vi "CS_Start.vi"() -> ()   [LabVIEW 2014]
doc: "\"Main\" of a CS system on the local machine. Mailny the SuperProc should be started from here. Other objects are created by the SuperProc itself. A list of names of all the objects to be created by the user is part of the data base (SuperProc->Special0-SpecialN).\n\nLicense Agreement for this software:\n\nCopyright (C) 2013 Holger Brand, Dennis Neidherr\nGSI Helmholtzzentrum für Schwerionenforschung GmbH\nPlanckstraße 1\nD-64291 Darmstadt\nGermany\n\nContact: d.neidherr@gsi.de \n\nThis program is free software: you can redistribute it and/or modify it under the terms\nof the GNU General Public License as published by the Free Software Foundation, either\nversion 3 of the License, or (at your option) any later version.\n\nThis program is distributed in the hope that it will be useful, but WITHOUT ANY WARRANTY;\nwithout even the implied warranty of MERCHANTABILITY or FITNESS FOR A PARTICULAR PURPOSE.\nSee the GNU General Public License for more details.\n\nYou should have received a copy of the GNU General Public License along with this program.\nIf not, see <http://www.gnu.org/licenses/>.\n\nFor all questions and ideas contact: d.neidherr@gsi.de or h.brand@gsi.de\nLast update: 20-Mar-2013\n\nmenuHelpStart\nFile\n==\n- \"Shutdown\" gently exits the CS system by removing all objects\n- \"Exit\" unfriendly exits the CS system by exiting the application without removing of objects. \n\nTools\n===\n- \"UserGOG\" displays a generic object GUI (GOG) for on-line testing purposes by the user sitting in front of the computer. If you would like to routinely open a GOG when a CS system starts, please configure a dedicated GOG via the database and configure the SuperProc to create that GOG upon starting up the system.\n\n- \"Inspector\" shows information on the objects of THIS and other CS systems.\n\n- \"DIM Table\" provides a simple possibility for viewing DIM services.\n\n- \"DIM Trend\" can be used for trending of DIM services\n\n- \"DIM Histogram\" can be used for histogramming of multiple DIM services\n\n- \"Access Viewer\" can be used to view the hierarchy of reserved objects. Moreover, it allows for locking the access to certain objects and sub-systems.\n\n- \"DSC Alarm Viewer\" is the alarm viewer of the SCADA backend based on the LabVIEW DSC module. When using the alarm viewer, you will be asked for the name of the DSC interface. The alarm viewer requires a binary compiled with the CSDSC_SCADA package.\nmenuHelpStop\n\ndescriptionHelpStart\n\"Main\" of a CS instance. CS is a framework that can be used by many experiments. CS is a multi-threaded, event driven, object oriented and distributed framework with SCADA functionality. An experiment control system can be developed by combining the CS framework with experiment specific add-ons.\n\nMore information available at http://wiki.gsi.de/cgi-bin/view/CSframework\n\ndescriptionHelpStop"
uses:
  CSClass/CSCore/GUIs/GOGFrontPanel/GOGFrontPanel.i attribute.ctl
  CSClass/CSCore/BaseProcess/BaseProcess.descriptor string definition.ctl
  CSClass/CSCore/CSSystem/CSSystemLib/CSSystemLib.instances options.ctl
  CSlibraries-extern/DimLVEvent/LVDimInterface/LVDimInterface.dim service type.ctl
  CSlibraries/UtilityLib/UtilityLib.helpType.ctl
  CSClass/CSCore/CSSystem/CoreDefs/CoreDefs.error_severity.ctl
  CSClass/CSCore/CSSystem/CoreDefs/CoreDefs.error_type.ctl
  CSlibraries/UtilityLib/UtilityLib.valueStatus.ctl
  CSlibraries-extern/DimLVEvent/LVDimInterface/LVDimInterface.dic_info_service_notifier.vi
  CSClass/CSCore/CSSystem/CoreLib/CoreLib.lvlib
  CSlibraries-extern/DimLVEvent/LVDimInterface/LVDimInterface.lvlib
  CSClass/CSCore/CSSystem/CSSystemLib/CSSystemLib.lvlib
  CSClass/CSCore/BaseProcess/BaseProcess.lvlib
  CSlibraries/UtilityLib/UtilityLib.lvlib
  CSClass/CSCore/CSObj/CSObj.lvlib
  CSClass/CSCore/CAEObj/CAEObj.lvlib
  CSClass/CSCore/BaseSM/BaseSM.lvlib
  CSClass/CSCore/BaseGUI/BaseGUI.lvlib
  CSClass/CSCore/GUIs/GOGFrontPanel/GOGFrontPanel.lvlib
panel:
  in  "False":bool
  out "database":string="Process@"
  out "domainInfo":string="hello world :-)"
  in  "GOGFrontPanel.i attribute":T1
  out "system running":bool=TRUE
  out "status":string="shutting down..."
  out "systemID":string="TestSystem@KSTest@lxgs11.gsi.de"
  out "error out":errorcluster
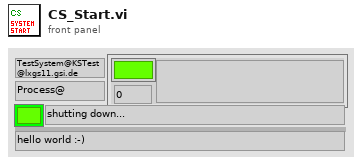
[diagram p1: front panel]
types:
  T1 = typedef "GOGFrontPanel.lvlib/GOGFrontPanel.i attribute.ctl" = cluster{"GOGObject":string, "Object":string, "Method":string, "Descriptor":T2, "Input Descriptor":string, "Output Descriptor":string, "inputNames":string[], "outputNames":string[], "Values":cluster{"descriptor":string, "value":string}[]}
  T2 = typedef "BaseProcess.lvlib/BaseProcess.descriptor string definition.ctl" = string
  T3 = enum32{"Invalid", "Standard", "Closed", "Hidden", "Minimized", "Maximized"}
  T4 = enum32{"invalid app kind", "Development System", "Run Time System", "Student Edition", "Embedded LabVIEW", "Evaluation", "Custom"}
  T5 = typedef "CSSystemLib.lvlib/CSSystemLib.instances options.ctl" = enum16{"add", "delete", "name2ref", "ref2name ", "ref2class", "obj exists?", "cleanup", "get I list", "get I list all", "ref2myclasses", "setClassNames"}
  T6 = enum16{"acquire queue", "release queue", "destroy queue", "get command ID", "destroy all queues"}
  T7 = typedef "UtilityLib.lvlib/UtilityLib.helpType.ctl" = enum16{"unknown", "menu", "description", "about", "special0", "special1", "special2"}
  T8 = typedef "CoreDefs.error_type.ctl" = enum16{"no error", "can't load process", "can't unload process", "process does not exist", "can't install process", "can't remove process", "unknown function", "time out", "can't execute function", "duplicate queue name", "super not found", "caller queue invalid", "can't ping process", "unknown error", "VISA Error", "VISA timeout", "GPIB timeout", "GPIB error", "communication error", "data type mismatch", "can't read data from OPC server", "can't write data to OPC server", "OET error", "function not implemented", "process already exists", "invalid Shared Variable name", "error writing Shared Variable", "error reading Shared Variable", "invalid client name", "corrupt database", "unknown class", "call not authorized", "parameter out of range", "OET timeout: can't get data to modify", "invalid queue name", "requested operation incompatible with current state", "event undefined", "event disabled", "state undefined", "caller is not a friend", "EventBuilder: bad eventID", "EventBuilder: no DAQ devices", "a thread must not stop itself", "UNUSED ELEMENT4", "DiscArchiver: eventData incomplete", "DiscArchiver: eventData does not belong to run", "DiscArchiver: can't open file", "DiscArchiver: can't write to file", "DiscArchiver: available disc space low", "can't acquire semaphore", "error reading data from database", "notifier object is not existing", "can't register process", "can't unregister process", "illegal event type", "object disabled", "object already exists", "can't change state", "Instrument not found", "no connection to remote node", "invalid reference", "N/A", "UNUSED ELEMENT 1", "element not found", "illegal TCP/IP connection detected", "object does not exist", "invalid access ID", "unknown CS system", "invalid privilige", "unsupported data type", "unsupported server type", "IO server already exists", "Shared Variable already exists"}
  T9 = typedef "CoreDefs.error_severity.ctl" = enum16{"undefined", "information", "warning", "error", "fatal"}
  T10 = typedef "UtilityLib.lvlib/UtilityLib.valueStatus.ctl" = enum16{"no info available", "stand by/off", "on", "warning", "alarm/malfunction", "not implemented", "user action required", "important information", "system default", "control default", "indicator default", "button default"}
  T11 = enum32{"Bad", "Idle", "Run top level", "Running"}
  T12 = typedef "LVDimInterface.lvlib/LVDimInterface.dim service type.ctl" = u16
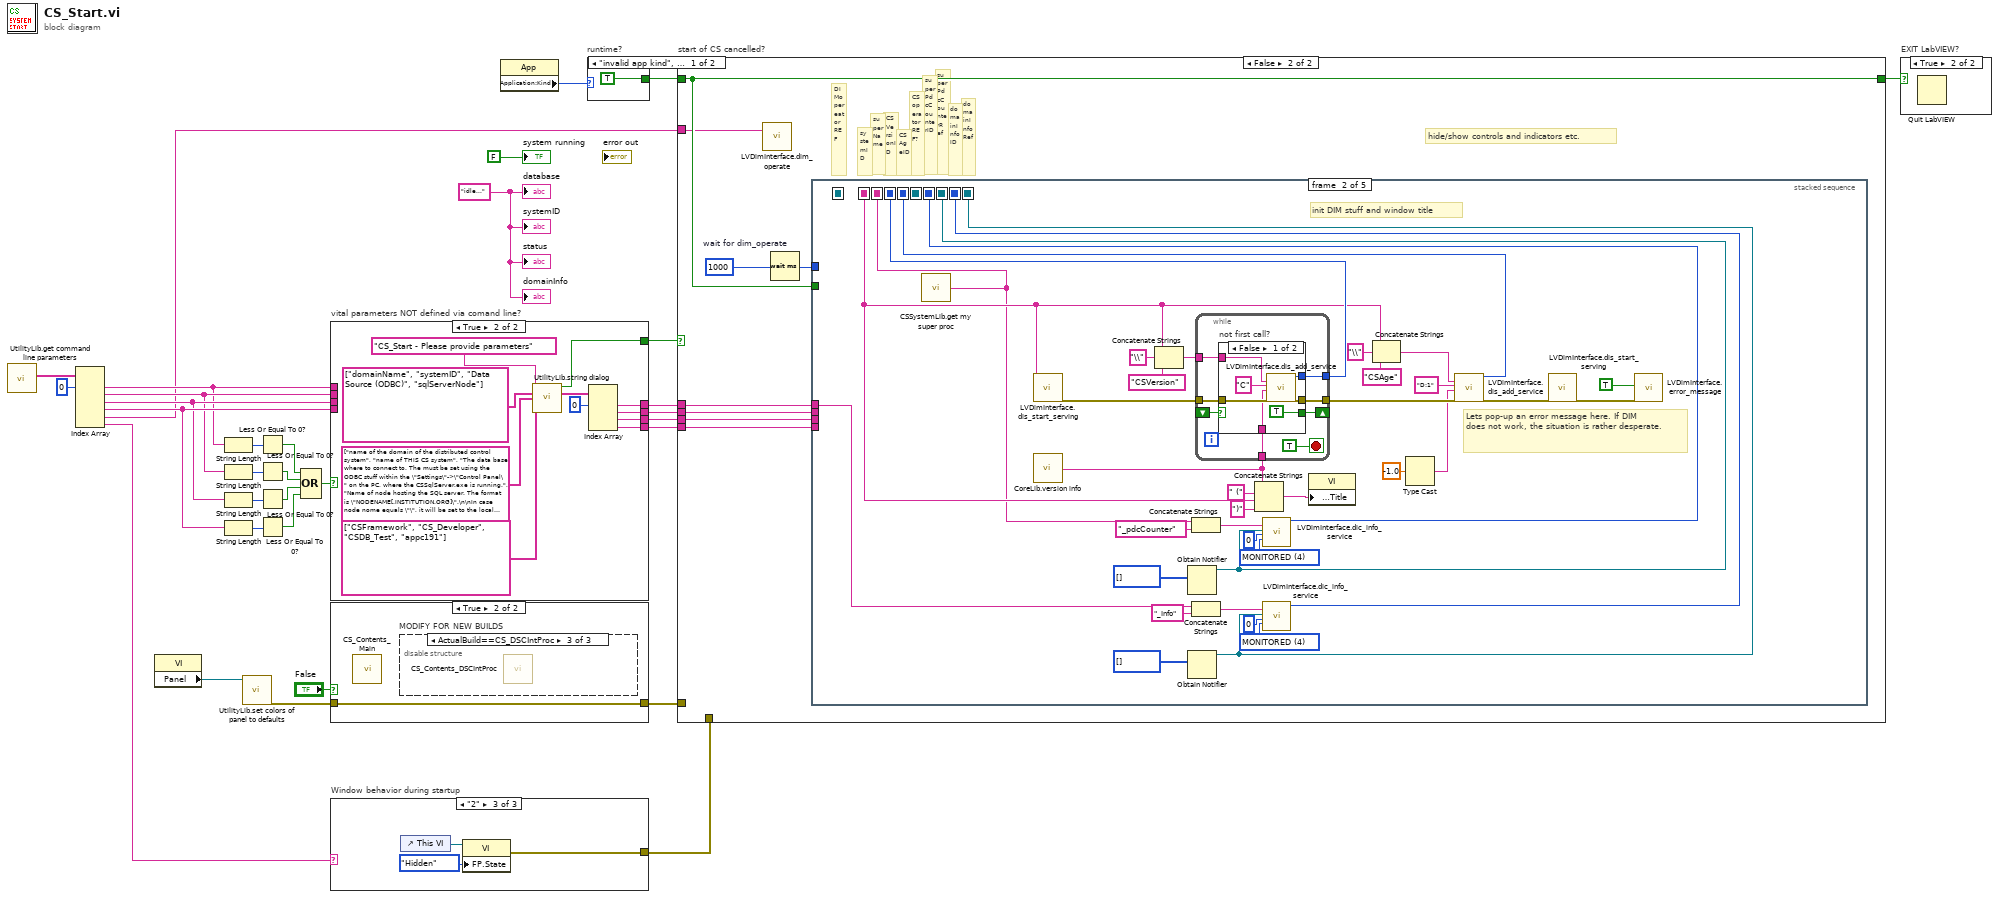
[diagram p0: block diagram]
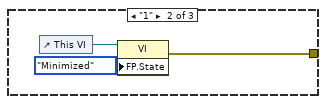
[diagram p3: hidden frame]
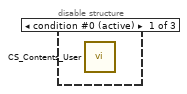
[diagram p5: hidden frame]
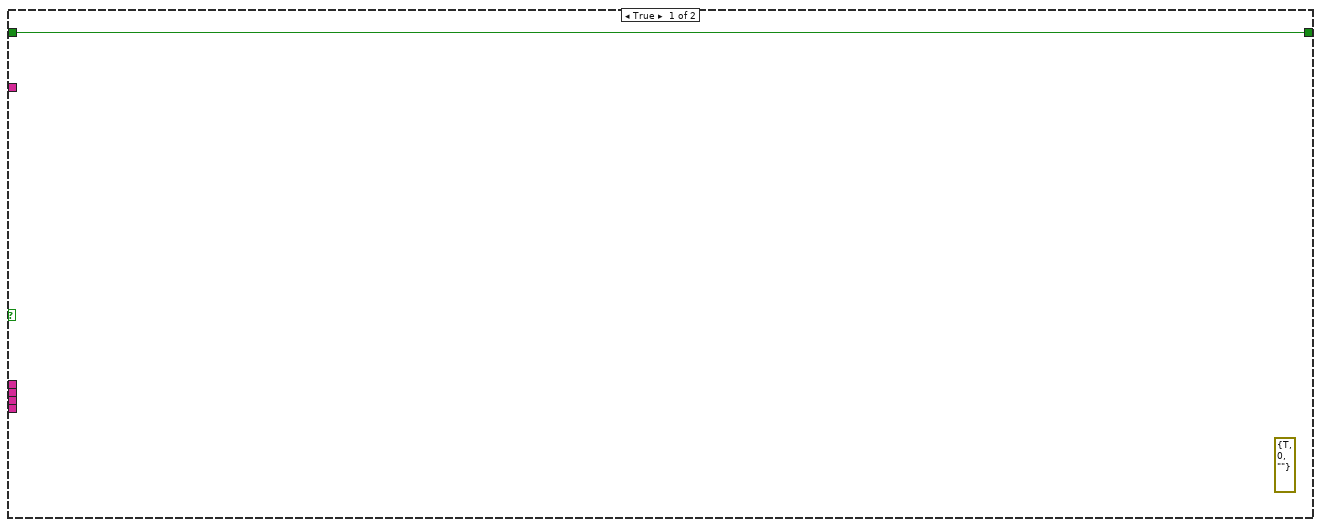
[diagram p8: hidden frame]
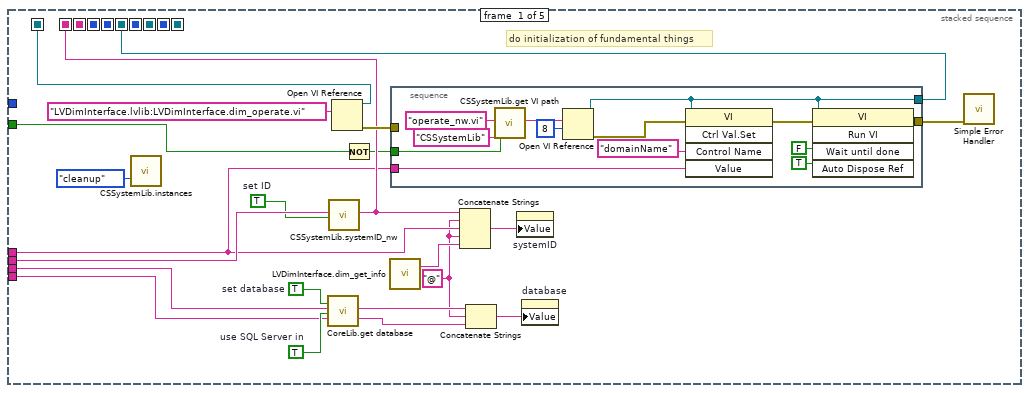
[diagram p9: hidden frame]
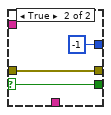
[diagram p10: hidden frame]
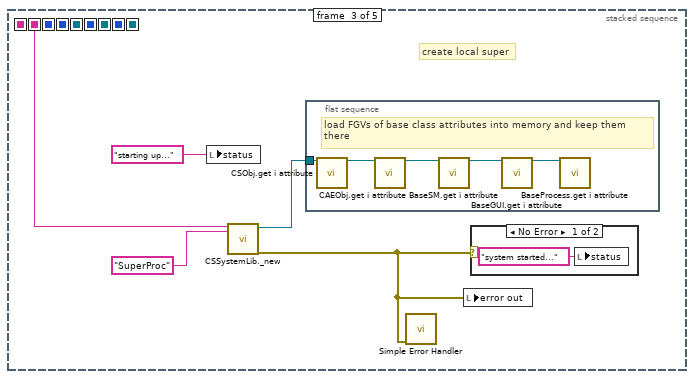
[diagram p11: hidden frame]
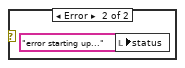
[diagram p12: hidden frame]
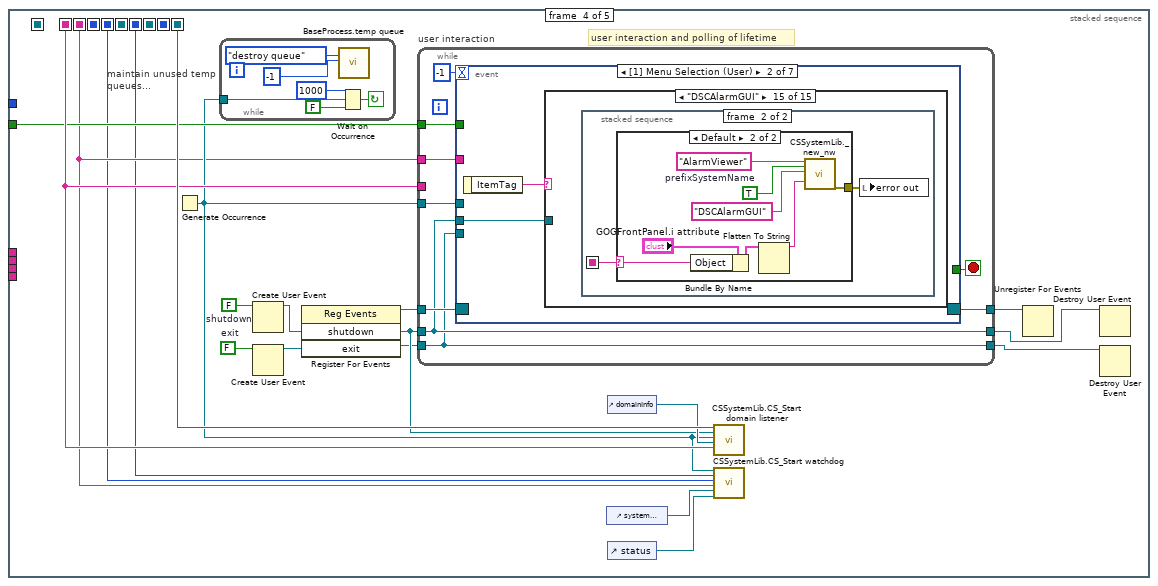
[diagram p13: hidden frame]
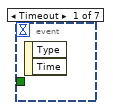
[diagram p14: hidden frame]
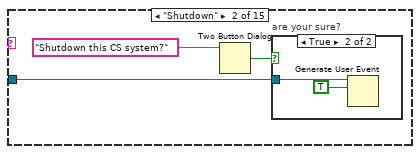
[diagram p16: hidden frame]
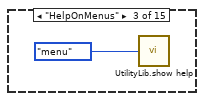
[diagram p18: hidden frame]
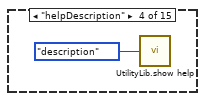
[diagram p19: hidden frame]
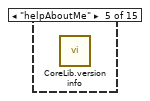
[diagram p20: hidden frame]
diagram:
  w10 = "idle..." ("status")
  n1 = call "UtilityLib.get command line parameters.vi"() -> ("parametersCleaned"=w30:string[])  [unwired: 9 in, 2 out]
  n2 = Index Array(array=w30, index #1=0 ("index")) -> (element #1=w18:string, element #2=w20:string, element #3=w22:string, element #4=w29:string, element #5=w5:string, element #6=w2:string)  [unwired: 5 in]
  n3 = property class="VI"() -> ("Panel"=w6:refnum<vi>)  [unwired: 2 in, 2 out]
  n4 = String Length(string=w18) -> (length=w17:i32)
  n5 = String Length(string=w20) -> (length=w19:i32)
  n6 = String Length(string=w22) -> (length=w21:i32)
  n7 = String Length(string=w29) -> (length=w27:i32)
  n8 = call "UtilityLib.set colors of panel to defaults.vi"("Front Panel"=w6) -> ("error out"=w9:errorcluster)  [unwired: 18 in]
  n9 = Less Or Equal To 0?(x=w17) -> (x <= 0?=w23:bool)
  n10 = Less Or Equal To 0?(x=w19) -> (x <= 0?=w24:bool)
  n11 = Less Or Equal To 0?(x=w21) -> (x <= 0?=w25:bool)
  n12 = Less Or Equal To 0?(x=w27) -> (x <= 0?=w28:bool)
  n13 = Compound Arithmetic op=OR(w23, w24, w25, w28) -> (w26:bool)
  n14 = case "vital parameters NOT defined via comand line?" shown="True" w26 {
    tunnel: [w36 w42] -> w14
    tunnel: w18 -> [w36 _]
    tunnel: [w35 w40] -> w1
    tunnel: w20 -> [w35 _]
    tunnel: w22 -> [w34 _]
    tunnel: [w34 w41] -> w13
    tunnel: w29 -> [w33 _]
    tunnel: [w33 w38] -> w12
    tunnel: [_ w39] -> w3
    frame False {
    }
    frame True {
      n15 = call "UtilityLib.string dialog.vi"("title"="CS_Start - Please provide parameters", "captions"=string[] ["domainName", "systemID", "Data Source (ODBC)", "sqlServerNode"], "helpText"=string[] ["name of the domain of the distributed control system", "name of THIS CS system", "The data base where to connect to. The must be set using the ODBC stuff within the \"Settings\"->\"Control Panel\" on the PC, where the CSSqlServer.exe is running.", "Name of node hosting the SQL server. The format is \"NODENAME[.INSTITUTION.ORG]\".\n\nIn case node nome equals \"\", it will be set to the local host."], "initialValue"=string[] ["CSFramework", "CS_Developer", "CSDB_Test", "appc191"]) -> ("cancelled"=w39:bool, "strings"=w44:string[])  [unwired: 8 in, 2 out]
      n16 = Index Array(array=w44, index #1=0 ("index")) -> (element #1=w42:string, element #2=w40:string, element #3=w41:string, element #4=w38:string)  [unwired: 3 in]
    }
  }
  n17 = case shown="True" "False" {
    tunnel: w9 -> [w48 w49]
    tunnel: [w48 w49] -> w8
    frame False {
    }
    frame True {
      n18 = call "CS_Contents_Main.vi"() -> ()  [unwired: 1 in]
      n19 = disable-structure "MODIFY FOR NEW BUILDS" shown="ActualBuild==CS_DSCIntProc" {
        frame condition #0 (active) {
          n20 = call "CS_Contents_User.vi"() -> ()  [unwired: 1 in]
        }
        frame condition #1 {
        }
        frame condition #2 {
          n21 = call "CS_Contents_DSCIntProc.vi"() -> ()  [unwired: 1 in]
        }
      }
    }
  }
  n22 = case "Window behavior during startup" shown="\"2\"" w2 {
    tunnel: [_ w52 w53] -> w4
    frame Default {
    }
    frame "1" {
      n23 = control-ref of="This VI"() -> (w50:refnum<vi>)
      n24 = property class="VI"(reference=w50, "FP.State"=T3."Minimized" ("Front Panel Window:State")) -> (error out=w52:errorcluster)  [unwired: 1 in, 1 out]
    }
    frame "2" {
      n25 = control-ref of="This VI"() -> (w55:refnum<vi>)
      n26 = property class="VI"(reference=w55, "FP.State"=T3."Hidden" ("Front Panel Window:State")) -> (error out=w53:errorcluster)  [unwired: 1 in, 1 out]
    }
  }
  n27 = property class="App"() -> ("Application:Kind"=w32:T4)  [unwired: 2 in, 2 out]
  n28 = case "runtime?" shown="\"invalid app kind\", Default" w32 {
    tunnel: [TRUE _] -> w16
    frame "invalid app kind", Default {
    }
    frame "Development System" {
    }
  }
  n29 = case "start of CS cancelled?" shown="False" w3 {
    tunnel: w16 -> [w57 w65]
    tunnel: [w57 w65] -> w15
    tunnel: w5 -> [_ w64]
    tunnel: w14 -> [_ w63]
    tunnel: w1 -> [_ w62]
    tunnel: w13 -> [_ w61]
    tunnel: w12 -> [_ w60]
    tunnel: w8 -> [_ _]
    tunnel: w4 -> [_ _]
    frame True {
      (unwired) errorcluster {"status"=TRUE, "code"=0, "source"=""} ("error out")
    }
    frame False {
      # "hide/show controls and indicators etc."
      # "domainInfoRef"
      # "domainInfoID"
      # "superPdcCounterRef"
      # "superPdcCounterID"
      # "CSoperator REF?"
      # "CSAgeID"
      # "CSVersionID"
      # "superName"
      # "systemID"
      # "DIMopereator REF"
      n30 = call "LVDimInterface.dim_operate.vi"("DNSNode"=w64) -> ()  [unwired: 19 in]
      n31 = Wait (ms) "wait for dim_operate"(milliseconds to wait=u32 1000) -> (millisecond timer value=w58:u32)
      n32 = stacked-sequence {
        seq-local: [w78 _ _ _ _] -> [_ w117 _ w184 _]
        seq-local: [w85 _ _ _ _] -> [_ _ _ _ w299]
        seq-local: [_ w109 _ _ _] -> [_ _ w158 w177 _]
        seq-local: [_ w126 _ _ _] -> [_ _ _ _ w295]
        seq-local: [_ w125 _ _ _] -> [_ _ _ w173 w294]
        seq-local: [w86 _ _ _ _] -> [_ _ _ _ w298]
        seq-local: [_ w113 _ _ _] -> [_ _ _ w174 w292]
        seq-local: [_ w112 _ _ _] -> [_ _ _ _ w290]
        seq-local: [_ w103 _ _ _] -> [_ _ _ _ w284]
        seq-local: [_ w102 _ _ _] -> [_ _ _ w185 w283]
        tunnel: w65 -> [w67 _ _ w180 w282]
        tunnel: w63 -> [w76 w101 _ _ _]
        tunnel: w62 -> [w77 _ _ _ _]
        tunnel: w61 -> [w81 _ _ _ _]
        tunnel: w60 -> [w80 _ _ _ _]
        tunnel: w58 -> [_ _ _ _ _]
        frame #0 {
          w74 = "@" ("string")
          w84 = TRUE  # use SQL Server in
          w87 = TRUE  # set database
          w66 = TRUE  # set ID
          # "do initialization of fundamental things"
          n33 = call "CSSystemLib.instances.vi"("Action"=CSSystemLib.instances_options."cleanup") -> ()  [unwired: 12 in, 7 out]
          n34 = call "CoreLib.get database.vi"("set database"=w87, "database in"=w81, "use SQL Server in"=w84, "SQL Server node in"=w80) -> ("database"=w75:string, "SQL Server node"=w73:string)  [unwired: 12 in, 2 out]
          n35 = call "CSSystemLib.systemID_nw.vi"("systemID"=w77, "Force set ID"=w66) -> ("systemID out"=w78:string)  [unwired: 16 in, 1 out]
          n36 = Open VI Reference(vi path="LVDimInterface.lvlib:LVDimInterface.dim_operate.vi") -> (vi reference=w85:refnum<vi>, error out=w82:errorcluster)  [unwired: 5 in]
          n37 = Not(x=w67) -> (.not. x?=w68:bool)
          n38 = call "LVDimInterface.dim_get_info.vi"() -> ("dimDnsNode"=w79:string)  [unwired: 13 in, 6 out]
          n39 = stacked-sequence {
            tunnel: w76 -> [w92]
            tunnel: [w96] -> w86
            tunnel: [w95] -> w69
            tunnel: w82 -> [_]
            tunnel: w68 -> [w89]
            frame #0 {
              n40 = call "CSSystemLib.get VI path.vi"("method"="operate_nw.vi" ("Method"), "class"="CSSystemLib" ("Class"), "reReead"=w89) -> ("VI path"=w91:string)  [unwired: 14 in, 2 out]
              n41 = Open VI Reference(vi path=w91, options=8) -> (vi reference=w96:refnum<vi>, error out=w99:errorcluster)  [unwired: 4 in]
              n42 = invoke class="VI" method="Ctrl Val.Set"(reference=w96, error in=w99, "Control Name"="domainName", "Value"=w92) -> (error out=w98:errorcluster)  [unwired: 1 in, 4 out]
              n43 = invoke class="VI" method="Run VI"(reference=w96, error in=w98, "Wait until done"=FALSE, "Auto Dispose Ref"=TRUE ("Auto Dispose Reference")) -> (error out=w95:errorcluster)  [unwired: 1 in, 4 out]
            }
          }
          n44 = Concatenate Strings(w78, w74, w76, w74, w79) -> (w72:string)
          n45 = Concatenate Strings(w75, w74, w73) -> (w71:string)
          n46 = property on="systemID" class="Str"("Value"=w72) -> ()  [unwired: 2 in, 2 out]
          n47 = property on="database" class="Str"("Value"=w71) -> ()  [unwired: 2 in, 2 out]
          n48 = call <vilib>:"Simple Error Handler.vi"("error in (no error)"=w69) -> ()  [unwired: 4 in, 5 out]
        }
        frame #1 {
          w108 = T12 4 items=["ONCE_ONLY"=1, "TIMED"=2, "MONITORED"=4] ("serviceType")
          w110 = T12 4 items=["ONCE_ONLY"=1, "TIMED"=2, "MONITORED"=4] ("serviceType")
          # "Lets pop-up an error message here. If DIM\ndoes not work, the situation is rather desperate."
          # "init DIM stuff and window title"
          n49 = call "CSSystemLib.get my super proc.vi"() -> ("name"=w109:string)  [unwired: 1 in]
          n50 = call "LVDimInterface.dis_start_serving.vi"("serverName"=w117) -> ("error out"=w134:errorcluster)  [unwired: 17 in, 1 out]
          n51 = call "CoreLib.version info.vi"() -> ("CS Version"=w121:string)  [unwired: 4 in, 1 out]
          n52 = Concatenate Strings(w117, "\\" ("string"), "CSVersion" ("string")) -> (w137:string)
          n53 = Obtain Notifier(notification data type=i8[] []) -> (notifier out=w112:refnum<notifier>)  [unwired: 3 in, 2 out]
          n54 = Obtain Notifier(notification data type=i8[] []) -> (notifier out=w102:refnum<notifier>)  [unwired: 3 in, 2 out]
          n55 = Concatenate Strings(w109, "_pdcCounter" ("string")) -> (w115:string)
          n56 = Concatenate Strings(w101, "_Info" ("string")) -> (w105:string)
          n57 = while {
            tunnel: w137 -> [w145]
            tunnel: w134 -> [w144]
            tunnel: [w143] -> w130
            tunnel: [w142] -> w126
            tunnel: w121 -> [w141]
            shift-right: [w139] -> _
            shift-left: _ -> [w138]
            stop <- TRUE stop-if-true
            n58 = case "not first call?" shown="False" w138 {
              selector: w138 -> [_ w153]
              tunnel: w145 -> [w152 _]
              tunnel: w144 -> [w150 w155]
              tunnel: [w149 w155] -> w143
              tunnel: [w148 -1 ("my_serviceID")] -> w142
              tunnel: w141 -> [w147 _]
              tunnel: [TRUE w153] -> w139
              frame False {
                n59 = call "LVDimInterface.dis_add_service.vi"("serviceName"=w152, "typeDescriptor"="C", "data"=w147, "error in (no error)"=w150) -> ("my_serviceID"=w148:i32, "error out"=w149:errorcluster)  [unwired: 14 in]
              }
              frame True {
              }
            }
          }
          n60 = Concatenate Strings(w121, " (" ("string"), w117, ")" ("string")) -> (w124:string)
          n61 = call-poly "LVDimInterface.dic_info_service.vi"("serviceName"=w115, "notifierRef"=w112, "timeout [s]"=0, "serviceType"=w110) -> ("callBackID"=w113:i32)  [unwired: 14 in, 1 out]
          n62 = call-poly "LVDimInterface.dic_info_service.vi"("serviceName"=w105, "notifierRef"=w102, "timeout [s]"=0, "serviceType"=w108) -> ("callBackID"=w103:i32)  [unwired: 14 in, 1 out]
          n63 = property class="VI"("Front Panel Window:Title"=w124) -> ()  [unwired: 2 in, 2 out]
          n64 = Concatenate Strings(w117, "\\" ("string"), "CSAge" ("string")) -> (w133:string)
          n65 = Type Cast(x=-1.0) -> (*(type *) &x=w128:string)  [unwired: 1 in]
          n66 = call "LVDimInterface.dis_add_service.vi"("serviceName"=w133, "typeDescriptor"="D:1", "data"=w128, "error in (no error)"=w130) -> ("my_serviceID"=w125:i32, "error out"=w119:errorcluster)  [unwired: 14 in]
          n67 = call "LVDimInterface.dis_start_serving.vi"("error in (no error)"=w119) -> ("error out"=w118:errorcluster)  [unwired: 17 in, 1 out]
          n68 = call "LVDimInterface.error_message.vi"("add message to source"=TRUE, "error in (no error)"=w118) -> ()  [unwired: 14 in, 4 out]
        }
        frame #2 {
          # "create local super"
          n69 = local write "status"("starting up..." ("status")) -> ()
          n70 = call "CSSystemLib._new.vi"("object name"=w158, "class name"="SuperProc") -> ("i ref out"=w157:refnum<vi>, "error out"=w156:errorcluster)  [unwired: 14 in, 2 out]
          n71 = flat-sequence {
            tunnel: w157 -> [w165]
            frame #0 {
              # "load FGVs of base class attributes into memory and keep them\nthere"
              n72 = call "CSObj.get i attribute.vi"("i ref in"=w165) -> ("i ref out"=w164:refnum<vi>)  [unwired: 16 in, 2 out]
              n73 = call "CAEObj.get i attribute.vi"("i ref in"=w164) -> ("i ref out"=w163:refnum<vi>)  [unwired: 16 in, 2 out]
              n74 = call "BaseSM.get i attribute.vi"("i ref in"=w163) -> ("i ref out"=w162:refnum<vi>)  [unwired: 16 in, 2 out]
              n75 = call "BaseGUI.get i attribute.vi"("i ref in"=w162) -> ("i ref out"=w161:refnum<vi>)  [unwired: 16 in, 2 out]
              n76 = call "BaseProcess.get i attribute.vi"("i ref in"=w161) -> ()  [unwired: 16 in, 3 out]
            }
          }
          n77 = call <vilib>:"Simple Error Handler.vi"("error in (no error)"=w156) -> ()  [unwired: 4 in, 5 out]
          n78 = local write "error out"(w156) -> ()
          n79 = case shown="No Error" w156 {
            frame No Error {
              n80 = local write "status"("system started..." ("status")) -> ()
            }
            frame Error {
              n81 = local write "status"("error starting up..." ("status")) -> ()
            }
          }
        }
        frame #3 {
          w171 = FALSE  # exit
          w172 = FALSE  # shutdown
          # "user interaction and polling of lifetime"
          n82 = Generate Occurrence() -> (w178:refnum<k4>)
          n83 = while "maintain unused temp queues..." {
            tunnel: w178 -> [w189]
            stop <- w190 continue-if-true
            n84 = Wait on Occurrence(1:FALSE ("ignore previous (T)"), 2:w189, 3:1000 ("ms timeout (-1)")) -> (0:w190:bool)
            n85 = call "BaseProcess.temp queue.vi"("Action"=T6."destroy queue", "ID in"=-1) -> ()  [unwired: 14 in, 4 out]
          }
          n86 = Create User Event(user event datatype=w172) -> (user event=w170:refnum<user-event>)  [unwired: 1 in, 1 out]
          n87 = Create User Event(user event datatype=w171) -> (user event=w169:refnum<user-event>)  [unwired: 1 in, 1 out]
          n88 = register-events(w170, w169) -> (reference out=w183:refnum<event-registration>)  [unwired: 2 in, 1 out]
          n89 = while "user interaction" {
            tunnel: w178 -> [w200]
            tunnel: w177 -> [w198]
            tunnel: w184 -> [_]
            tunnel: w180 -> [w196]
            tunnel: w183 -> [w195]
            tunnel: w170 -> [w194]
            tunnel: [w193] -> w182
            tunnel: [w194] -> w168
            tunnel: w169 -> [w192]
            tunnel: [w192] -> w181
            stop <- w199 stop-if-true
            n90 = event shown="[1] Menu Selection (User)" {
              selector: w195 -> [_ _ _ _ _ _ _]
              dyn-events: [_ _ _ _ _ _ _] -> w193
              timeout: -1 -> [_ _ _ _ _ _ _]
              tunnel: w200 -> [_ _ _ w265 _ _ _]
              tunnel: w198 -> [_ _ _ w264 _ _ _]
              tunnel: [_ _ _ w263 _ _ _] -> w199
              tunnel: w196 -> [_ _ _ _ _ _ w277]
              tunnel: w194 -> [_ w201 _ _ _ _ _]
              tunnel: w192 -> [_ _ _ _ w272 w276 _]
              event Timeout {
                n91 = event-data() -> ()  [unwired: 1 in, 2 out]
              }
              event Menu Selection (User) {
                n92 = event-data() -> ("ItemTag"=w202:string)  [unwired: 1 in]
                n93 = case shown="\"DSCAlarmGUI\"" w202 {
                  tunnel: w201 -> [_ w203 _ _ _ _ _ _ _ _ _ _ _ _ _]
                  frame Default {
                  }
                  frame "Shutdown" {
                    n94 = Two Button Dialog(message="Shutdown this CS system?") -> (T button?=w204:bool)  [unwired: 2 in]
                    n95 = case "are your sure?" shown="True" w204 {
                      tunnel: w203 -> [_ w206]
                      frame False {
                      }
                      frame True {
                        n96 = Generate User Event(user event=w206, event data cluster=TRUE ("event data")) -> ()  [unwired: 2 in, 2 out]
                      }
                    }
                  }
                  frame "HelpOnMenus" {
                    n97 = call "UtilityLib.show help.vi"("helpType"=UtilityLib.helpType."menu") -> ()
                  }
                  frame "helpDescription" {
                    n98 = call "UtilityLib.show help.vi"("helpType"=UtilityLib.helpType."description") -> ()
                  }
                  frame "helpAboutMe" {
                    n99 = call "CoreLib.version info.vi"() -> ()  [unwired: 4 in, 2 out]
                  }
                  frame "helpExplainError" {
                    n100 = call "CoreLib.explain error.vi"() -> ()  [unwired: 1 in]
                  }
                  frame "ApplicationInfo" {
                    n101 = property class="App"() -> ("App.Name"=w212:string, "App.Version"=w210:string)  [unwired: 2 in, 2 out]
                    n102 = Concatenate Strings("name: " ("string"), w212, ", version: " ("string"), w210) -> (w214:string)
                    n103 = One Button Dialog(message=w214) -> ()  [unwired: 1 in, 1 out]
                  }
                  frame "UserGOG" {
                    w218 = TRUE  # prefixSystemName
                    n104 = call "CSSystemLib._new_nw.vi"("objectName"="UserGOG", "prefixSystemName"=w218, "className"="GeneralObjectGUI", "data in"="N/A") -> ("error out"=w217:errorcluster)  [unwired: 13 in, 2 out]
                    n105 = local write "error out"(w217) -> ()
                  }
                  frame "Inspector" {
                    w223 = TRUE  # prefixSystemName
                    n106 = call "CSSystemLib._new_nw.vi"("objectName"="Inspector" ("Data"), "prefixSystemName"=w223, "className"="ObjectInspector", "data in"="N/A") -> ("error out"=w222:errorcluster)  [unwired: 13 in, 2 out]
                    n107 = local write "error out"(w222) -> ()
                  }
                  frame "DIMTable" {
                    w228 = TRUE  # prefixSystemName
                    n108 = call "CSSystemLib._new_nw.vi"("objectName"="DIMTable" ("Data"), "prefixSystemName"=w228, "className"="DIMTableView", "data in"="N/A") -> ("error out"=w227:errorcluster)  [unwired: 13 in, 2 out]
                    n109 = local write "error out"(w227) -> ()
                  }
                  frame "DIMTrendGUI" {
                    w233 = TRUE  # prefixSystemName
                    n110 = call "CSSystemLib._new_nw.vi"("objectName"="DIMTrend" ("Data"), "prefixSystemName"=w233, "className"="DIMTrendGUI", "data in"="N/A") -> ("error out"=w232:errorcluster)  [unwired: 13 in, 2 out]
                    n111 = local write "error out"(w232) -> ()
                  }
                  frame "DIMHistogramGUI" {
                    w238 = TRUE  # prefixSystemName
                    n112 = call "CSSystemLib._new_nw.vi"("objectName"="DIMHistogram" ("Data"), "prefixSystemName"=w238, "className"="DIMHistogramGUI", "data in"="N/A") -> ("error out"=w237:errorcluster)  [unwired: 13 in, 2 out]
                    n113 = local write "error out"(w237) -> ()
                  }
                  frame "ToolsDispatchMessageBox" {
                    n114 = call "CSSystemLib.CS_Start dispatch message box.vi"() -> ("error out"=w240:errorcluster)  [unwired: 18 in, 1 out]
                    n115 = local write "error out"(w240) -> ()
                  }
                  frame "AccessViewer" {
                    w244 = TRUE  # prefixSystemName
                    n116 = call "CSSystemLib._new_nw.vi"("objectName"="AccessViewer" ("Data"), "prefixSystemName"=w244, "className"="CSAccessViewer", "data in"="N/A") -> ("error out"=w243:errorcluster)  [unwired: 13 in, 2 out]
                    n117 = local write "error out"(w243) -> ()
                  }
                  frame "DSCAlarmGUI" {
                    n118 = stacked-sequence {
                      seq-local: [w246 _] -> [_ w248]
                      frame #0 {
                        n119 = call "CSSystemLib._getInstances_nw.vi"() -> ("i list"=w247:string[])  [unwired: 18 in, 1 out]
                        n120 = call "UtilityLib.selectName.vi"("names"=w247) -> ("name"=w246:string)  [unwired: 16 in, 2 out]
                      }
                      frame #1 {
                        n121 = case shown="Default" w248 {
                          selector: w248 -> [_ w253]
                          tunnel: [w252 w258] -> w249
                          frame "" {
                            n122 = call "CoreLib.my to LV error.vi"("ErrorTypes"=CoreDefs.error_type."process does not exist", "severityLevel"=CoreDefs.error_severity."information") -> ("myErrorCluster"=w252:errorcluster)  [unwired: 16 in, 1 out]
                          }
                          frame Default {
                            w259 = TRUE  # prefixSystemName
                            n123 = Bundle By Name(cluster="GOGFrontPanel.i attribute", "Object"=w253) -> (w255:T1)
                            n124 = Flatten To String(anything=w255) -> (data string=w254:string)  [unwired: 3 in, 2 out]
                            n125 = call "CSSystemLib._new_nw.vi"("objectName"="AlarmViewer" ("Data"), "prefixSystemName"=w259, "className"="DSCAlarmGUI", "data in"=w254) -> ("error out"=w258:errorcluster)  [unwired: 13 in, 2 out]
                          }
                        }
                        n126 = local write "error out"(w249) -> ()
                      }
                    }
                  }
                }
              }
              event "domainInfo": Mouse Down {
                n127 = event-data() -> ()  [unwired: 1 in, 1 out]
                n128 = control-ref of="domainInfo"() -> (w262:refnum<vi>)
                n129 = call "UtilityLib.set color of simple string or numeric.vi"("simpleString"=w262, "valueStatus"=UtilityLib.valueStatus."indicator default") -> ()  [unwired: 17 in, 1 out]
              }
              event User Event {
                n130 = event-data() -> ("shutdown"=w263:bool)  [unwired: 1 in]
                n131 = case "shutdown?" shown="True" w263 {
                  tunnel: w264 -> [_ w270]
                  tunnel: w265 -> [_ w268]
                  frame False {
                  }
                  frame True {
                    n132 = Set Occurrence(w268) -> ()
                    n133 = call "CSSystemLib.name2ref.vi"("name"=w270) -> ("obj refnum"=w267:refnum<vi>)
                    n134 = call "CSSystemLib._delete.vi"("i ref"=w267) -> ("error out"=w266:errorcluster)  [unwired: 18 in]
                    n135 = property on="error out" class="Clust (strict)"("Value"=w266) -> ()  [unwired: 2 in, 2 out]
                    n136 = local write "status"("shutting down..." ("status")) -> ()
                  }
                }
              }
              event Panel Close? {
                n137 = event-data() -> ()  [unwired: 1 in, 1 out]
                n138 = Generate User Event(user event=w272, event data cluster=TRUE ("event data")) -> ()  [unwired: 2 in, 2 out]
                n139 = event-data("Discard?"=TRUE) -> ()  [unwired: 1 in, 1 out]
              }
              event Application Instance Close? {
                n140 = event-data() -> ()  [unwired: 1 in, 1 out]
                n141 = Generate User Event(user event=w276, event data cluster=TRUE ("event data")) -> ()  [unwired: 2 in, 2 out]
                n142 = event-data("Discard?"=TRUE) -> ()  [unwired: 1 in, 1 out]
              }
              event User Event {
                n143 = event-data() -> ()  [unwired: 1 in, 1 out]
                n144 = Two Button Dialog(message="Exit this CS system without shutdown?") -> (T button?=w278:bool)  [unwired: 2 in]
                n145 = case "exit CS?" shown="False" w277 {
                  tunnel: w278 -> [_ w281]
                  frame False {
                    n146 = One Button Dialog(message="\"EXIT\" is not available in the development system. ") -> ()  [unwired: 1 in, 1 out]
                  }
                  frame True {
                    n147 = case "Exit application?" shown="True" w281 {
                      frame False {
                      }
                      frame True {
                        n148 = Quit LabVIEW() -> ()  [unwired: 1 in]
                      }
                    }
                  }
                }
              }
            }
          }
          n149 = control-ref of="system running"() -> (w176:refnum<vi>)
          n150 = control-ref of="domainInfo"() -> (w179:refnum<vi>)
          n151 = control-ref of="status"() -> (w175:refnum<vi>)
          n152 = call "CSSystemLib.CS_Start domain listener.vi"("domainInfo"=w185, "shutdown"=w170, "stop"=w178, "domainInfoDisplay"=w179, "systemID"=w184) -> ()  [unwired: 15 in]
          n153 = call "CSSystemLib.CS_Start watchdog.vi"("stop"=w178, "superPdcCounterID"=w174, "CSAgeID"=w173, "superName"=w177, "systemRunning"=w176, "status"=w175) -> ()  [unwired: 14 in]
          n154 = Unregister For Events(event registration refnum=w182) -> ()  [unwired: 1 in, 1 out]
          n155 = Destroy User Event(user event=w168) -> ()  [unwired: 1 in, 1 out]
          n156 = Destroy User Event(user event=w181) -> ()  [unwired: 1 in, 1 out]
        }
        frame #4 {
          # "shut down DIM stuff"
          n157 = flat-sequence {
            tunnel: [w305] -> w289
            frame #0 {
              n158 = call "BaseProcess.temp queue.vi"("Action"=T6."destroy all queues") -> ()  [unwired: 15 in, 4 out]
              n159 = call "CSSystemLib.updateInstanceList_nw.vi"("remove list"=TRUE) -> ()  [unwired: 4 in]
            }
            frame #1 {
              n160 = call "LVDimInterface.dis_start_serving.vi"("serverName"="dummy") -> ("error out"=w305:errorcluster)  [unwired: 17 in, 1 out]
            }
          }
          n161 = call "LVDimInterface.dic_release_service.vi"("callBackID"=w284) -> ("error out"=w286:errorcluster)  [unwired: 18 in]
          n162 = call "LVDimInterface.dic_release_service.vi"("callBackID"=w292) -> ("error out"=w291:errorcluster)  [unwired: 18 in]
          n163 = case shown="False" FALSE ("Case Constant\n(See Context Help)") {
            tunnel: [_ w301] -> w296
            tunnel: w295 -> [_ w300]
            frame False {
            }
            frame True {
              # "always keep\none service!"
              n164 = call "LVDimInterface.dis_remove_service.vi"("my_serviceID"=w300) -> ("error out"=w301:errorcluster)  [unwired: 18 in]
            }
          }
          n165 = Release Notifier(notifier=w283, error in (no error)=w286) -> (error out=w285:errorcluster)  [unwired: 1 in, 2 out]
          n166 = Release Notifier(notifier=w290, error in (no error)=w291) -> (error out=w287:errorcluster)  [unwired: 1 in, 2 out]
          n167 = call "LVDimInterface.dis_remove_service.vi"("my_serviceID"=w294, "error in (no error)"=w296) -> ("error out"=w293:errorcluster)  [unwired: 17 in]
          n168 = case "runtime system?" shown="False" w282 {
            tunnel: w299 -> [w310 w323]
            tunnel: w298 -> [w307 w324]
            tunnel: [w307 w324] -> w297
            tunnel: w293 -> [_ _]
            tunnel: w289 -> [_ _]
            tunnel: w287 -> [_ _]
            tunnel: w285 -> [_ _]
            frame False {
              n169 = flat-sequence {
                tunnel: w310 -> [w312]
                tunnel: [w312] -> w309
                tunnel: w307 -> [w311]
                tunnel: w309 -> [w319]
                frame #0 {
                  n170 = while {
                    tunnel: w311 -> [w317]
                    stop <- w315 stop-if-true
                    n171 = property class="VI"(reference=w317) -> ("Execution:State"=w316:T11)  [unwired: 1 in, 2 out]
                    n172 = Less Or Equal?(x=w316, y=T11."Idle" ("Execution:State")) -> (x <= y?=w315:bool)
                    n173 = Wait Until Next ms Multiple(millisecond multiple=u32 250) -> ()  [unwired: 1 out]
                  }
                }
                frame #1 {
                  n174 = invoke class="VI" method="Ctrl Val.Set"(reference=w319, "Control Name"="stop", "Value"=TRUE) -> (error out=w320:errorcluster)  [unwired: 2 in, 4 out]
                  n175 = Close Reference(reference=w319, error in (no error)=w320) -> ()  [unwired: 1 out]
                }
              }
              n176 = invoke class="VI" method="Ctrl Val.Set"(reference=w307, "Control Name"="stop", "Value"=TRUE) -> ()  [unwired: 2 in, 5 out]
            }
            frame True {
              n177 = flat-sequence {
                tunnel: w323 -> [w325]
                tunnel: [w325] -> w322
                tunnel: w322 -> [w326]
                frame #0 {
                  n178 = call "LVDimInterface.dis_stop_serving.vi"() -> ()  [unwired: 19 in, 1 out]
                }
                frame #1 {
                  n179 = invoke class="VI" method="Ctrl Val.Set"(reference=w326, "Control Name"="stop", "Value"=TRUE) -> ()  [unwired: 2 in, 5 out]
                }
              }
            }
          }
          n180 = Close Reference(reference=w297) -> ()  [unwired: 1 in, 1 out]
        }
      }
    }
  }
  n181 = case "EXIT LabVIEW?" shown="True" w15 {
    frame False {
    }
    frame True {
      n182 = Quit LabVIEW() -> ()  [unwired: 1 in]
    }
  }
  "status" <- w10
  "domainInfo" <- w10
  "system running" <- FALSE ("system running")
  "systemID" <- w10
  "database" <- w10
